vi "Exercise.vi"() -> ()   [LabVIEW 2014]
uses:
  <vilib>/measure/NI_MABase.lvlib
panel:
  in  "Delay":u32
  in  "stop":bool
  out "Waveform Chart":dbl(graph)
  in  "sampling info":cluster{"Fs":dbl, "#s":dbl}={"Fs"=1000.0, "#s"=1000.0} {"Fs" format="%.2p"}
  in  "phase":dbl format="%.2p"
  in  "amplitude":dbl=1.0 format="%0.2p"
  in  "frequency":dbl=10.0 format="%0.2p"
  in  "signal type":T1(ring)
  in  "offset":dbl format="%0.2p"
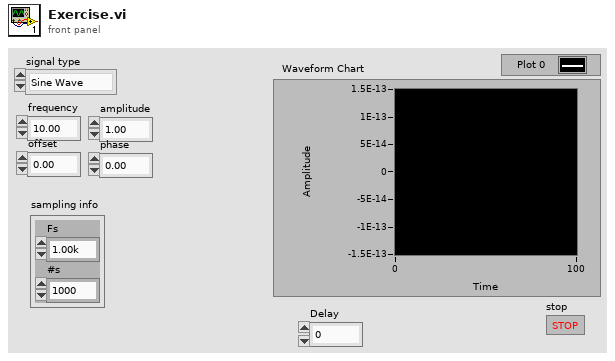
[diagram p1: front panel]
types:
  T1 = enum16{"Sine Wave", "Triangle Wave", "Square Wave", "Sawtooth Wave"}
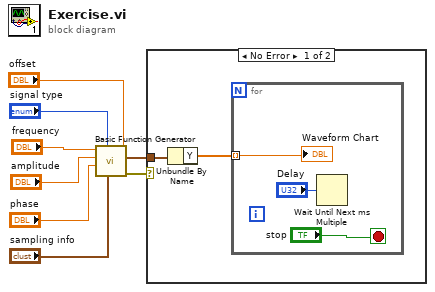
[diagram p0: block diagram]
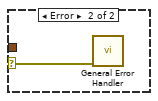
[diagram p2: hidden frame]
diagram:
  n1 = call <vilib>:"Basic Function Generator.vi"("offset"="offset", "sampling info"="sampling info", "signal type"="signal type", "phase"="phase", "amplitude"="amplitude", "frequency"="frequency") -> ("error out"=w8:errorcluster, "signal out"=w7:waveform(dbl))  [unwired: 3 in, 1 out]
  n2 = case shown="No Error" w8 {
    selector: w8 -> [_ w14]
    tunnel: w7 -> [w10 _]
    frame No Error {
      n3 = Unbundle By Name(w10) -> ("Y"=w9:dbl[])
      n4 = for {
        tunnel: w9 -> [w13] mode=indexing
        stop <- "stop" stop-if-true
        n5 = Wait Until Next ms Multiple(millisecond multiple="Delay") -> ()  [unwired: 1 out]
        "Waveform Chart" <- w13
      }
    }
    frame Error {
      n6 = call <vilib>:"General Error Handler.vi"("error in (no error)"=w14) -> ()  [unwired: 10 in, 5 out]
    }
  }
